vi "Write Step.vi"(8 "error in (no error)":errorcluster, 10 "Step":i32, 11 "Fortress In":refnum<class "Fortress.lvclass">) -> (0 "error out":errorcluster, 3 "Fortress Out":refnum<class "Fortress.lvclass">)   [LabVIEW 2015, in "Fortress.lvclass"]
uses:
  Fortress.lvclass
  Fortress.lvclass/Fortress.ctl
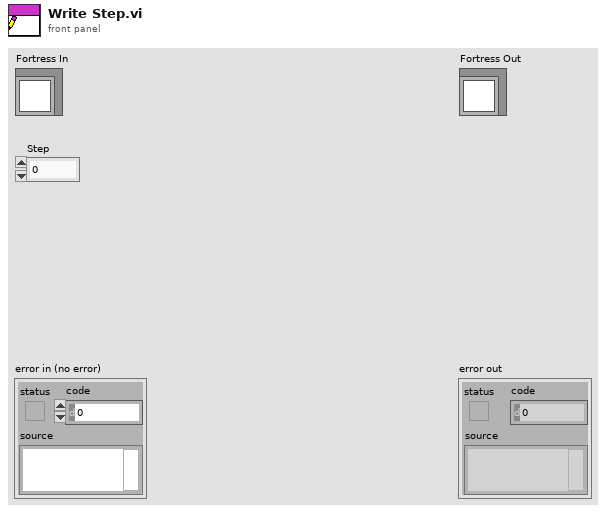
[diagram p1: front panel]
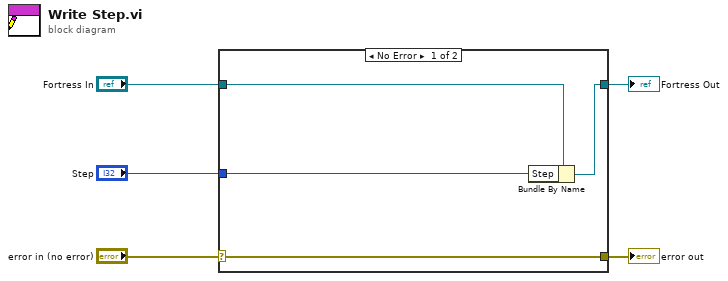
[diagram p0: block diagram]
diagram:
  n1 = case shown="No Error" "error in (no error)" {
    selector: "error in (no error)" -> [w9 w10]
    tunnel: [w9 w10] -> w4
    tunnel: [w7 w11] -> w2
    tunnel: "Fortress In" -> [w8 w11]
    tunnel: "Step" -> [w6 _]
    frame No Error {
      n2 = Bundle By Name(cluster=w8, "Step"=w6) -> (w7:refnum<class "Fortress.lvclass">)
    }
    frame Error {
    }
  }
  "error out" <- w4
  "Fortress Out" <- w2
